vi "oa_Compute DC Gap Value (N Channels).vi"(0 "scaled signal [EU]":waveform(dbl)[](array[waveform]), 1 "reset?":bool, 3 "select reference data":T1(ring), 7 "start points":dbl[](array[numeric]), 9 "durations":dbl[](array[numeric]), 11 "error in":errorcluster, 12 "averaging type":enum16{"Linear", "Exponential"}(ring), 14 "window":T2(ring)) -> (4 "DC out":dbl[](array[numeric]), 15 "error out":errorcluster)   [LabVIEW 2017, in "SoundVib_RefDataProcess.lvlib"]
uses:
  <vilib>/addons/Sound and Vibration/Order Analysis/Referece Data Processing/SoundVib_RefDataProcess.lvlib
  <vilib>/measure/madcrms.llb/Basic Averaged DC-RMS for 1 Chan.vi
  <vilib>/Waveform/WDTOps.llb/WDT Get Waveform Subset DBL.vi
  <vilib>/measure/madcrms.llb/Basic Averaged DC-RMS for N Chan.vi
  <vilib>/measure/NI_MAPro.lvlib
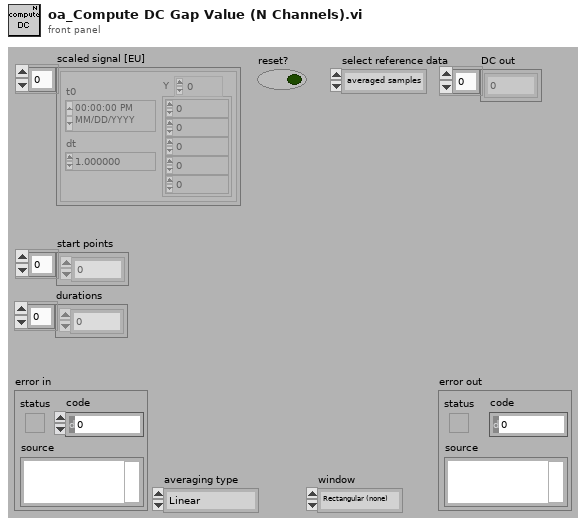
[diagram p1: front panel]
types:
  T1 = enum16{"averaged samples", "initial samples", "final samples"}
  T2 = enum16{"Rectangular (none)", "Hanning", "Low side lobe"}
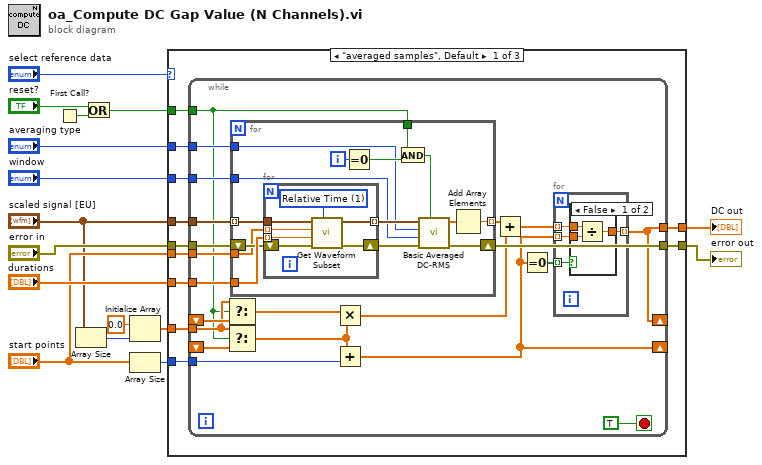
[diagram p0: block diagram]
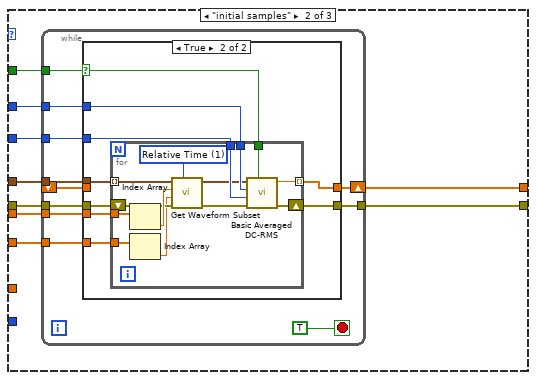
[diagram p3: hidden frame]
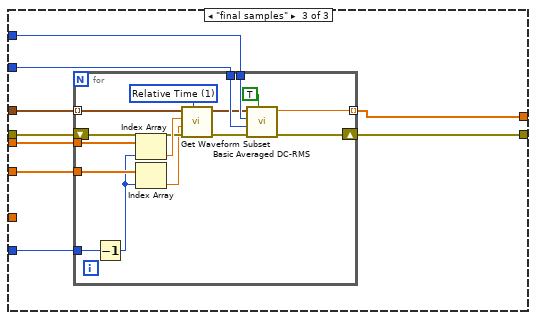
[diagram p5: hidden frame]
diagram:
  n1 = First Call?() -> (First Call?: T/F=w5:bool)
  n2 = Array Size(array="scaled signal [EU]") -> (size(s)=w3:i32)
  n3 = Or(x="reset?", y=w5) -> (x .or. y?=w6:bool)
  n4 = Initialize Array(0.0 ("element"), w3) -> (w1:dbl[])
  n5 = Array Size(array="start points") -> (size(s)=w8:i32)
  n6 = case shown="\"averaged samples\", Default" "select reference data" {
    tunnel: "start points" -> [w26 w83 w132]
    tunnel: "durations" -> [w25 w82 w126]
    tunnel: "scaled signal [EU]" -> [w24 w84 w128]
    tunnel: w6 -> [w27 w87 _]
    tunnel: "averaging type" -> [w22 w86 w130]
    tunnel: "window" -> [w21 w85 w129]
    tunnel: "error in" -> [w23 w81 w127]
    tunnel: [w17 w80 w124] -> w14
    tunnel: [w20 w79 w125] -> w16
    tunnel: w8 -> [w19 _ w131]
    tunnel: w1 -> [w18 _ _]
    frame "averaged samples", Default {
      n7 = while {
        tunnel: w27 -> [w35]
        tunnel: w26 -> [w47]
        tunnel: w25 -> [w46]
        tunnel: w24 -> [w45]
        tunnel: w23 -> [w38]
        tunnel: w22 -> [w44]
        tunnel: w21 -> [w43]
        tunnel: [w42] -> w20
        shift-right: [w37] -> _
        shift-left: _ -> [w41]
        shift-right: [w29] -> _
        shift-left: _ -> [w40]
        tunnel: [w37] -> w17
        tunnel: w19 -> [w36]
        tunnel: w18 -> [w39]
        stop <- TRUE stop-if-true
        n8 = Select(t=w39, s=w35, f=w41) -> (s? t:f=w34:dbl[])
        n9 = Select(t=w39, s=w35, f=w40) -> (s? t:f=w33:dbl[])
        n10 = for {
          tunnel: w47 -> [w68]
          tunnel: w46 -> [w70]
          tunnel: w45 -> [w71] mode=indexing
          shift-right: [w66] -> w42
          shift-left: w38 -> [w69]
          tunnel: w44 -> [w60]
          tunnel: w43 -> [w59]
          tunnel: w35 -> [w62]
          tunnel: [w57] -> w31 mode=indexing
          i -> [w64]
          n11 = for {
            tunnel: w71 -> [w78]
            tunnel: w70 -> [w77] mode=indexing
            tunnel: w68 -> [w74] mode=indexing
            shift-right: [w73] -> w67
            shift-left: w69 -> [w76]
            tunnel: [w72] -> w65 mode=indexing
            w75 = u16 1 items=["Index", "Relative Time"] ("Mode")
            n12 = call-poly <vilib>:"Get Waveform Subset.vi"("start/duration format"=w75, "error in (no error)"=w76, "duration"=w77, "start samples/time"=w74, "waveform in"=w78) -> ("error out"=w73:errorcluster, "waveform out"=w72:waveform(dbl))  [unwired: 1 in, 2 out]
          }
          n13 = Equal To 0?(x=w64) -> (x = 0?=w63:bool)
          n14 = And(x=w62, y=w63) -> (x .and. y?=w61:bool)
          n15 = call-poly <vilib>:"Basic Averaged DC-RMS.vi"("reset"=w61, "error in (no error)"=w67, "window"=w59, "averaging type"=w60, "signals in"=w65) -> ("error out"=w66:errorcluster, "DC values"=w58:dbl[])  [unwired: 3 in, 2 out]
          n16 = Add Array Elements(numeric array=w58) -> (sum=w57:dbl)
        }
        n17 = Multiply(x=w34, y=w33) -> (x*y=w30:dbl[])
        n18 = Add(x=w33, y=w36) -> (x+y=w29:dbl[])
        n19 = Add(x=w31, y=w30) -> (x+y=w32:dbl[])
        n20 = Equal To 0?(x=w29) -> (x = 0?=w28:bool[])
        n21 = for {
          tunnel: [w52] -> w37 mode=indexing
          tunnel: w32 -> [w51] mode=indexing
          tunnel: w29 -> [w50] mode=indexing
          tunnel: w28 -> [w49] mode=indexing
          n22 = case shown="False" w49 {
            tunnel: [w55 w56] -> w52
            tunnel: w51 -> [w54 w56]
            tunnel: w50 -> [w53 _]
            frame False {
              n23 = Divide(x=w54, y=w53) -> (x/y=w55:dbl)
            }
            frame True {
            }
          }
        }
      }
    }
    frame "initial samples" {
      n24 = while {
        tunnel: w87 -> [w91]
        tunnel: w86 -> [w98]
        tunnel: w85 -> [w97]
        tunnel: w84 -> [w96]
        tunnel: w83 -> [w95]
        tunnel: w82 -> [w94]
        tunnel: w81 -> [w93]
        shift-right: [w90] -> w80
        shift-left: _ -> [w89]
        tunnel: [w88] -> w79
        stop <- TRUE stop-if-true
        n25 = case shown="True" w91 {
          selector: w91 -> [_ w103]
          tunnel: w98 -> [_ w109]
          tunnel: w97 -> [_ w108]
          tunnel: w96 -> [_ w107]
          tunnel: w95 -> [_ w106]
          tunnel: w94 -> [_ w105]
          tunnel: w93 -> [w99 w104]
          tunnel: [w100 w102] -> w90
          tunnel: w89 -> [w100 _]
          tunnel: [w99 w101] -> w88
          frame False {
          }
          frame True {
            n26 = for {
              tunnel: w109 -> [w123]
              tunnel: w108 -> [w122]
              tunnel: w107 -> [w121] mode=indexing
              tunnel: w106 -> [w119]
              tunnel: w105 -> [w111]
              tunnel: w103 -> [w114]
              tunnel: [w113] -> w102 mode=indexing
              shift-right: [w112] -> w101
              shift-left: w104 -> [w117]
              w120 = u16 1 items=["Index", "Relative Time"] ("Mode")
              n27 = Index Array(array=w119) -> (element=w118:dbl)  [unwired: 1 in]
              n28 = Index Array(array=w111) -> (element=w110:dbl)  [unwired: 1 in]
              n29 = call-poly <vilib>:"Get Waveform Subset.vi"("start/duration format"=w120, "error in (no error)"=w117, "duration"=w110, "start samples/time"=w118, "waveform in"=w121) -> ("error out"=w116:errorcluster, "waveform out"=w115:waveform(dbl))  [unwired: 1 in, 2 out]
              n30 = call-poly <vilib>:"Basic Averaged DC-RMS.vi"("reset"=w114, "error in (no error)"=w116, "window"=w122, "averaging type"=w123, "signal in"=w115) -> ("error out"=w112:errorcluster, "DC value"=w113:dbl)  [unwired: 3 in, 2 out]
            }
          }
        }
      }
    }
    frame "final samples" {
      n31 = for {
        tunnel: w132 -> [w148]
        tunnel: w131 -> [w147]
        tunnel: w130 -> [w145]
        tunnel: w129 -> [w144]
        tunnel: w128 -> [w143] mode=indexing
        tunnel: w126 -> [w136]
        tunnel: [w137] -> w124 mode=indexing
        shift-right: [w138] -> w125
        shift-left: w127 -> [w140]
        w133 = u16 1 items=["Index", "Relative Time"] ("Mode")
        n32 = Decrement(x=w147) -> (x-1=w135:i32)
        n33 = Index Array(array=w148, index=w135) -> (element=w141:dbl)
        n34 = Index Array(array=w136, index=w135) -> (element=w134:dbl)
        n35 = call-poly <vilib>:"Get Waveform Subset.vi"("start/duration format"=w133, "error in (no error)"=w140, "duration"=w134, "start samples/time"=w141, "waveform in"=w143) -> ("error out"=w139:errorcluster, "waveform out"=w142:waveform(dbl))  [unwired: 1 in, 2 out]
        n36 = call-poly <vilib>:"Basic Averaged DC-RMS.vi"("reset"=TRUE, "error in (no error)"=w139, "window"=w144, "averaging type"=w145, "signal in"=w142) -> ("error out"=w138:errorcluster, "DC value"=w137:dbl)  [unwired: 3 in, 2 out]
      }
    }
  }
  "error out" <- w16
  "DC out" <- w14
